vi "test udp w.vi"() -> ()   [LabVIEW 2019]
uses:
  <vilib>/numeric/Random Number (Range) I64.vi
  <vilib>/numeric/sub_Random U32.vi
panel:
  out "에러 출력":errorcluster
  out "웨이브폼 그래프":i64[][](graph)
  in  "대기 시간 (ms)":u32
  out "출력 배열":u8[](array[numeric])
  out "배열":i64[][](array[numeric])
  in  "Stop":bool
  in  "dt":u32=50
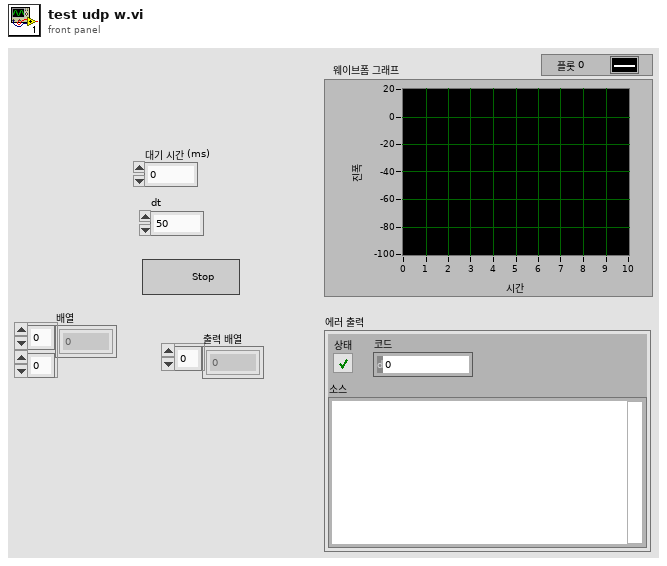
[diagram p1: front panel]
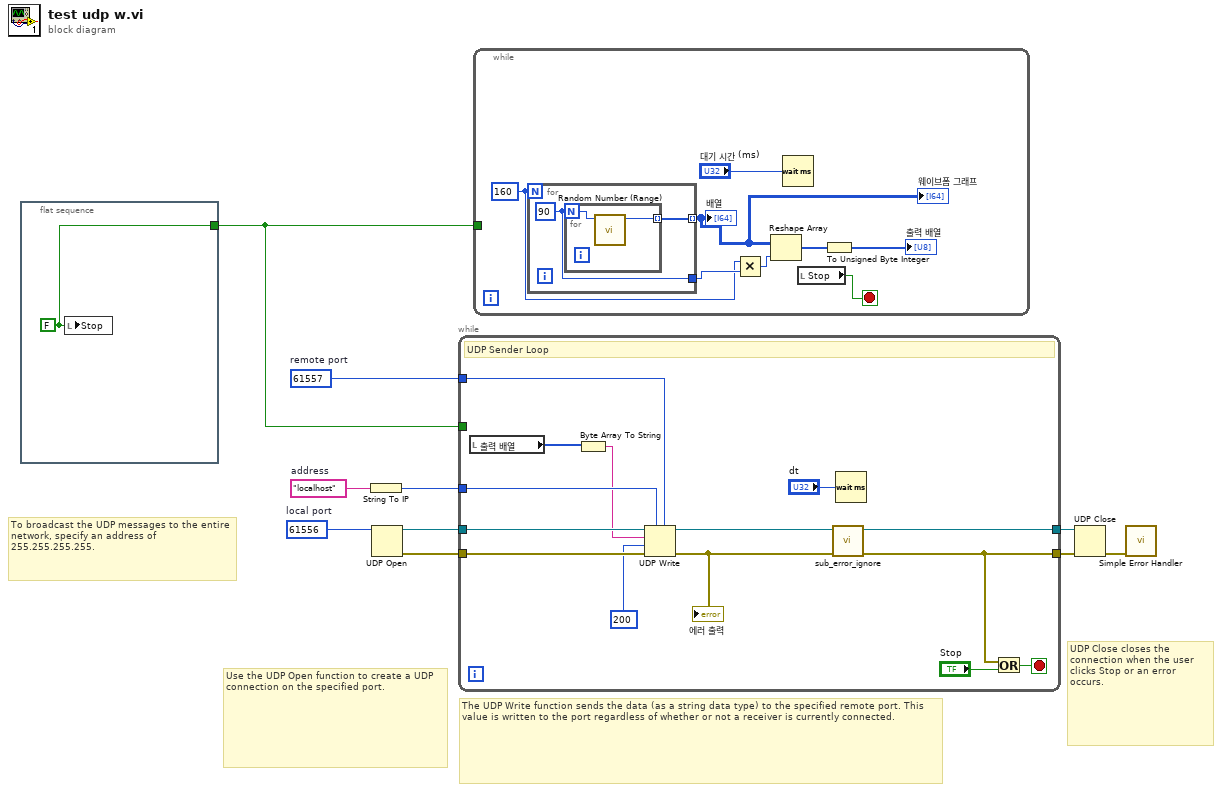
[diagram p0: block diagram]
diagram:
  w2 = u16 61557  # remote port
  w3 = u16 61556  # local port
  w8 = "localhost"  # address
  # "To broadcast the UDP messages to the entire network, specify an address of 255.255.255.255."
  # "UDP Close closes the connection when the user clicks Stop or an error occurs."
  # "The UDP Write function sends the data (as a string data type) to the specified remote port. This value is written to the port regardless of whether or not a receiver is currently connected."
  # "Use the UDP Open function to create a UDP connection on the specified port."
  n1 = flat-sequence {
    tunnel: [w11] -> w1
    frame #0 {
      w11 = FALSE ("Stop")
      n2 = local write "Stop"(w11) -> ()
    }
  }
  n3 = String To IP(1:w8) -> (0:w6:u32)
  n4 = UDP Open(11:w3) -> (port=w5:refnum<k16>, 0:w4:errorcluster)  [unwired: 4 in, 1 out]
  n5 = while {
    tunnel: [w14] -> w9
    tunnel: w5 -> [w24]
    tunnel: w4 -> [w23]
    tunnel: [w16] -> w10
    tunnel: w6 -> [w20]
    tunnel: w2 -> [w18]
    tunnel: w1 -> [_]
    stop <- w22 stop-if-true
    # "UDP Sender Loop"
    n6 = local read "출력 배열"() -> (w13:u8[])
    n7 = Byte Array To String(unsigned byte array=w13) -> (string=w12:string)
    n8 = UDP Write(address=w20, port or service name=w18, connection ID=w24, data in=w12, 8:w23, 9:200 ("타임아웃 ms (25000)")) -> (error out=w15:errorcluster, 3:w16:refnum<k16>)
    "에러 출력" <- w15
    n9 = call "sub_error_ignore.vi"("error in"=w15) -> ("error out"=w14:errorcluster)  [unwired: 10 in]
    n10 = Wait (ms)(milliseconds to wait="dt") -> ()  [unwired: 1 out]
    n11 = Or(x=w14, y="Stop") -> (x .or. y?=w22:bool)
  }
  n12 = while {
    tunnel: w1 -> [_]
    stop <- w28 stop-if-true
    w31 = 160
    n13 = for {
      N: w31 -> [_]
      tunnel: [w34] -> w26 mode=indexing
      tunnel: [w33] -> w32
      w33 = 90
      n14 = for {
        N: w33 -> [w36]
        tunnel: [w35] -> w34 mode=indexing
        n15 = call-poly <vilib>:"Random Number (Range).vi"("upper bound (100)"=w36) -> ("number"=w35:i64)  [unwired: 10 in]
      }
    }
    "배열" <- w26
    "웨이브폼 그래프" <- w26
    n16 = Multiply(x=w31, y=w32) -> (x*y=w30:i32)
    n17 = Reshape Array(w26, w30) -> (w29:i64[])
    n18 = Wait (ms)(milliseconds to wait="대기 시간 (ms)") -> ()  [unwired: 1 out]
    n19 = local read "Stop"() -> (w28:bool)
    n20 = To Unsigned Byte Integer(number=w29) -> (unsigned 8bit integer=→"출력 배열":u8[])
  }
  n21 = UDP Close(connection ID=w10, 8:w9) -> (error out=w7:errorcluster)  [unwired: 1 out]
  n22 = call <vilib>:"Simple Error Handler.vi"("error in (no error)"=w7) -> ()  [unwired: 4 in, 5 out]
